vi "Stop Core.vi"(10 "final error code":i32, 11 "Controller in":refnum<class "Controller.lvclass">) -> (3 "Controller out":refnum<class "Controller.lvclass">)   [LabVIEW 2011, in "Controller.lvclass"]
doc: "(<B>Filename</B>: Actor Framework.lvlib:Actor.lvclass:Stop Core.vi)\n\nDefines what the actor does before it stops. Use the <B>final error code</B> input to determine whether the actor shut down in response to an error.\n\nBy default, this method does nothing. A descendant class may override it to define behavior, such as shutting down any processes the actor initiated in its override of the Actor Core method."
uses:
  Controller.lvclass
  <userlib>/_Frameworks/ActorFramework/Actor/Actor.lvclass
  Controller.lvclass/Controller.ctl
  <userlib>/_Frameworks/ActorFramework/Message Enqueuer/Message Enqueuer.lvclass/Message Enqueuer.ctl
  <userlib>/_Frameworks/ActorFramework/Message Enqueuer/Enqueue.vi
  <userlib>/_Frameworks/ActorFramework/Message Priority Queue/Priority Enqueue.vi
  <userlib>/_Frameworks/ActorFramework/Stop Msg/Stop Msg.lvclass
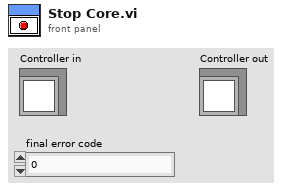
[diagram p1: front panel]
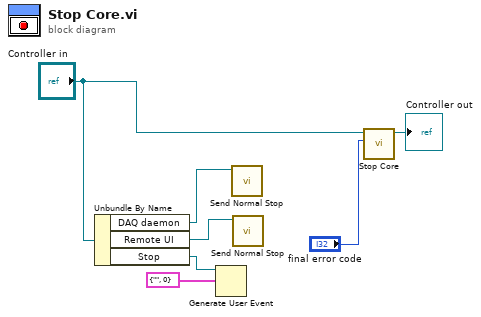
[diagram p0: block diagram]
diagram:
  n1 = Unbundle By Name("Controller in") -> ("DAQ daemon"=w2:refnum<class "Message Enqueuer.lvclass">, "Remote UI"=w1:refnum<class "Message Enqueuer.lvclass">, "Stop"=w5:refnum<user-event>)
  n2 = Generate User Event(user event=w5, event data cluster=cluster{string, i32} {"", 0} ("event data")) -> ()  [unwired: 1 in, 2 out]
  n3 = call <userlib>:"Send Normal Stop.vi"("Message Enqueuer"=w2) -> ()  [unwired: 10 in, 1 out]
  n4 = call <userlib>:"Send Normal Stop.vi"("Message Enqueuer"=w1) -> ()  [unwired: 10 in, 1 out]
  n5 = call-parent "Stop Core.vi"("final error code"="final error code", "Actor in"="Controller in") -> ("Actor out"=→"Controller out":refnum<class "Controller.lvclass">)  [unwired: 9 in]
